vi "update_RF_generators.vi"(8 "error in":errorcluster, 11 "GPIB (in)":refnum<class "GPIB.lvclass">) -> (0 "error out":errorcluster, 3 "GPIB":refnum<class "GPIB.lvclass">)   [LabVIEW 2013, in "GPIB.lvclass"]
uses:
  GPIB.lvclass
  GPIB.lvclass/GPIB.ctl
  HP83623A_RF_Generator/HP83623A_RF_Generator.lvclass
  HP83712B_RF_Generator/HP83712B_RF_Generator.lvclass
  HP8662A_RF_Generator/HP8662A_RF_Generator.lvclass
  Experiment/Globals.vi
  Experiment/Experiment.lvclass
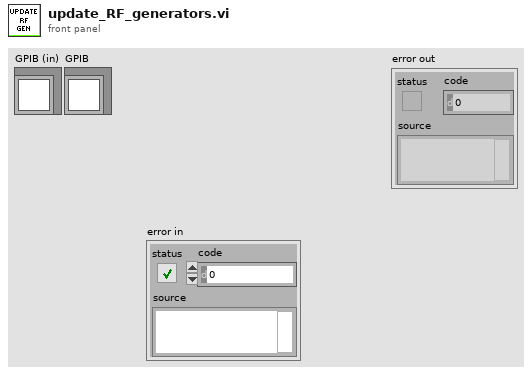
[diagram p1: front panel]
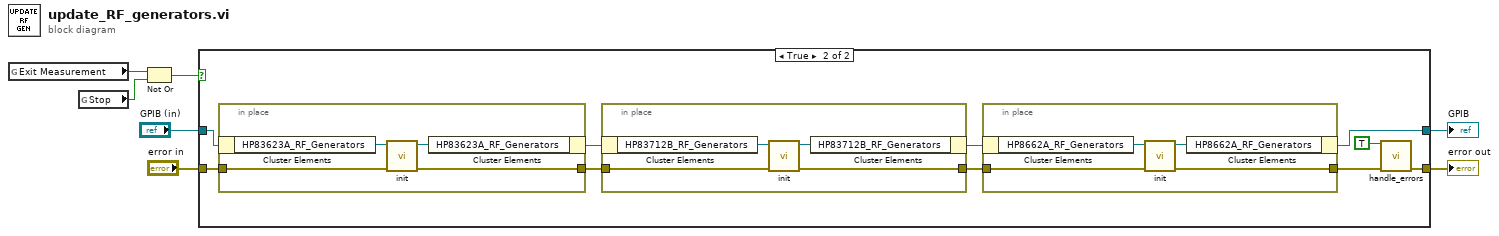
[diagram p0: block diagram]
diagram:
  n1 = global read "Globals.vi" "Exit Measurement"() -> (w3:bool)
  n2 = global read "Globals.vi" "Stop"() -> (w2:bool)
  n3 = Not Or(1:w2, 2:w3) -> (0:w1:bool)
  n4 = case shown="True" w1 {
    tunnel: "error in" -> [w8 w19]
    tunnel: "GPIB (in)" -> [w9 w18]
    tunnel: [w9 w14] -> w5
    tunnel: [w8 w11] -> w4
    frame False {
    }
    frame True {
      n5 = in-place {
        in-place-border: w19 -> [w31]
        in-place-border: [w28] -> w16
        n6 = in-place-cluster #1(w18) -> ("HP83623A_RF_Generators"=w30:refnum<class "HP83623A_RF_Generator.lvclass">)
        n7 = call-dynamic "init.vi"("error in (no error)"=w31, "HP83623A_RF_Generator in"=w30) -> ("error out"=w28:errorcluster, "HP83623A_RF_Generator out"=w29:refnum<class "HP83623A_RF_Generator.lvclass">)  [unwired: 8 in]
        n8 = in-place-cluster #1("HP83623A_RF_Generators"=w29) -> (w17:refnum<class "GPIB.lvclass">)
      }
      n9 = in-place {
        in-place-border: w16 -> [w25]
        in-place-border: [w24] -> w13
        n10 = in-place-cluster #2(w17) -> ("HP83712B_RF_Generators"=w27:refnum<class "HP83712B_RF_Generator.lvclass">)
        n11 = call-dynamic "init.vi"("error in (no error)"=w25, "HP83712B_RF_Generator in"=w27) -> ("error out"=w24:errorcluster, "HP83712B_RF_Generator out"=w26:refnum<class "HP83712B_RF_Generator.lvclass">)  [unwired: 8 in]
        n12 = in-place-cluster #2("HP83712B_RF_Generators"=w26) -> (w15:refnum<class "GPIB.lvclass">)
      }
      n13 = in-place {
        in-place-border: w13 -> [w23]
        in-place-border: [w20] -> w12
        n14 = in-place-cluster #3(w15) -> ("HP8662A_RF_Generators"=w22:refnum<class "HP8662A_RF_Generator.lvclass">)
        n15 = call-dynamic "init.vi"("error in (no error)"=w23, "HP8662A_RF_Generator in"=w22) -> ("error out"=w20:errorcluster, "HP8662A_RF_Generator out"=w21:refnum<class "HP8662A_RF_Generator.lvclass">)  [unwired: 8 in]
        n16 = in-place-cluster #3("HP8662A_RF_Generators"=w21) -> (w14:refnum<class "GPIB.lvclass">)
      }
      n17 = call "handle_errors.vi"("Exit Operation"=TRUE ("Exit Measurement"), "error in (no error)"=w12) -> ("error out"=w11:errorcluster)  [unwired: 13 in]
    }
  }
  "error out" <- w4
  "GPIB" <- w5
